vi "BUFMGR_set_maxmem.vi"(5 "megs in":u64, 11 "error in (no error)":errorcluster) -> (4 "return":u32 format="%.0x", 15 "error out":errorcluster)   [LabVIEW 2016]
uses:
  c/lib/libbuf.so
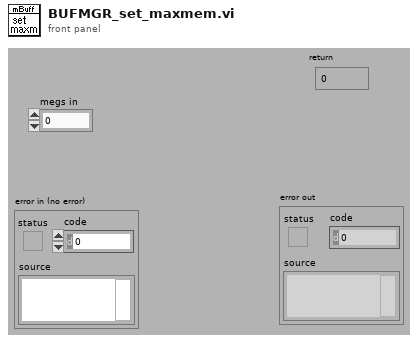
[diagram p1: front panel]
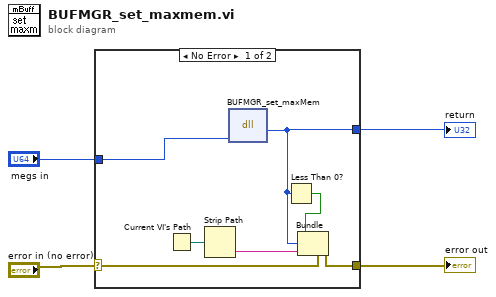
[diagram p0: block diagram]
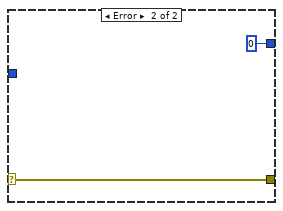
[diagram p2: hidden frame]
diagram:
  n1 = case shown="No Error" "error in (no error)" {
    selector: "error in (no error)" -> [w5 w12]
    tunnel: [w8 u32 0] -> w4
    tunnel: "megs in" -> [w11 _]
    tunnel: [w10 w12] -> w2
    frame No Error {
      n2 = Current VI's Path() -> (path=w7:path)
      n3 = Strip Path(path=w7) -> (name=w6:string)  [unwired: 1 out]
      n4 = dll-call lib="home/simager/panview/PAN/Modules/buffermgr/private/c/lib/libbuf.so" fn="BUFMGR_set_maxMem"("megs"=w11) -> ("return type"=w8:u32)  [unwired: 4 in, 2 out]
      n5 = Less Than 0?(x=w8) -> (x < 0?=w9:bool)
      n6 = Bundle(cluster=w5, "status"=w9, "code"=w8, "source"=w6) -> (w10:errorcluster)
    }
    frame Error {
    }
  }
  "error out" <- w2
  "return" <- w4
